vi "Scroll_Pump_Serial_Packet_Read.vi"(0 "VISA resource In":refnum<visa-resource-name>, 11 "error in":errorcluster) -> (4 "VISA resource Out":refnum<visa-resource-name>, 8 "Data Out":string, 15 "error out":errorcluster)   [LabVIEW 2014]
uses:
  <vilib>/Instr/_visa.llb/VISA Flush IO Buffer Mask.ctl
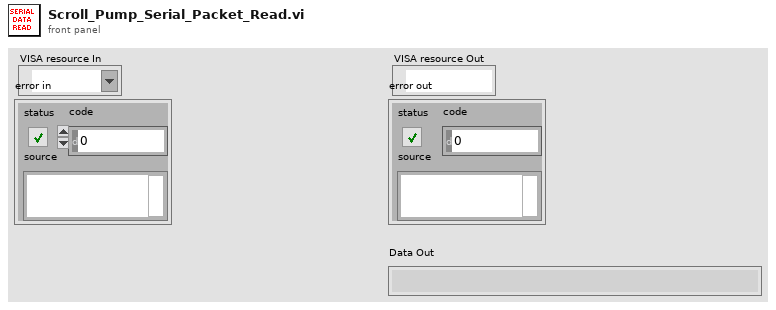
[diagram p1: front panel]
types:
  T1 = typedef "VISA Flush IO Buffer Mask.ctl" = u16
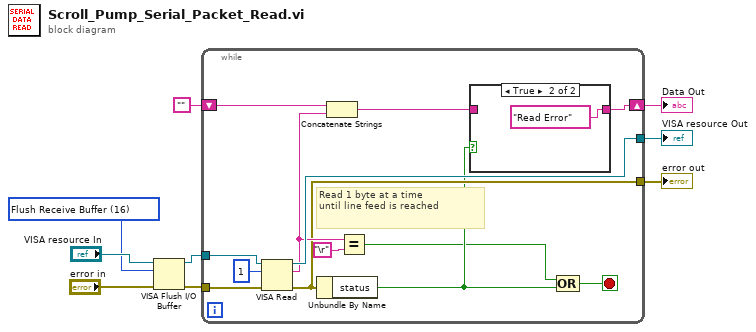
[diagram p0: block diagram]
diagram:
  w1 = T1 16 items=["Flush Receive Buffer"=16, "Write Transmit Buffer to Device"=32, "Flush Receive Buffer (No I/O)"=64, "Flush Transmit Buffer"=128] ("Mask")
  n1 = VISA Flush I/O Buffer(VISA resource name="VISA resource In", mask (16)=w1, error in (no error)="error in") -> (VISA resource name out=w5:refnum<visa-resource-name>, error out=w4:errorcluster)
  n2 = while {
    tunnel: [w22] -> w8
    tunnel: [w15] -> w7
    tunnel: w5 -> [w21]
    tunnel: w4 -> [w20]
    shift-right: [w13] -> w9
    shift-left: "" -> [w19]
    stop <- w10 stop-if-true
    # "Read 1 byte at a time \nuntil line feed is reached"
    n3 = VISA Read(VISA resource name=w21, byte count=u32 1, error in (no error)=w20) -> (VISA resource name out=w22:refnum<visa-resource-name>, read buffer=w18:string, error out=w15:errorcluster)  [unwired: 1 out]
    n4 = Unbundle By Name(w15) -> ("status"=w12:bool)
    n5 = Concatenate Strings(w19, w18) -> (w14:string)
    n6 = Equal?(x=w18, y="\r") -> (x = y?=w11:bool)
    n7 = case shown="True" w12 {
      tunnel: w14 -> [w23 _]
      tunnel: [w23 "Read Error"] -> w13
      frame False {
      }
      frame True {
      }
    }
    n8 = Compound Arithmetic op=OR(w11, w12) -> (w10:bool)
  }
  "VISA resource Out" <- w8
  "error out" <- w7
  "Data Out" <- w9
